vi "json_string_unescape.vi"(11 "escaped string":string) -> (2 "characters unescaped?":bool, 3 "string out":string)   [LabVIEW 2017]
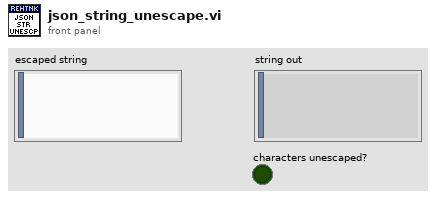
[diagram p1: front panel]
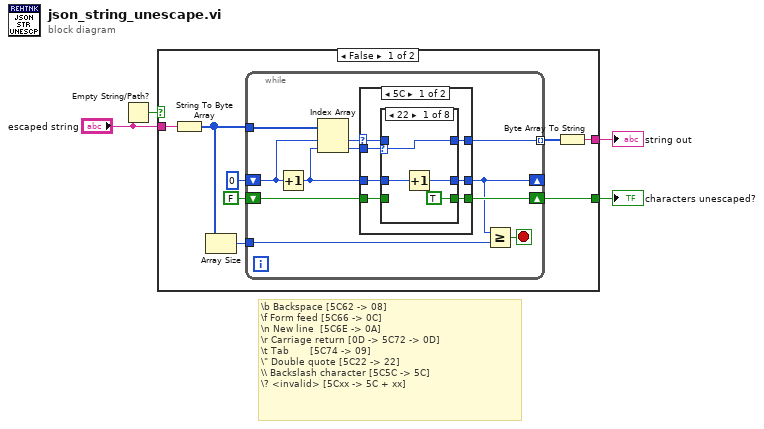
[diagram p0: block diagram]
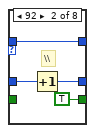
[diagram p2: hidden frame]
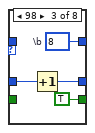
[diagram p3: hidden frame]
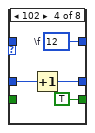
[diagram p4: hidden frame]
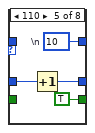
[diagram p5: hidden frame]
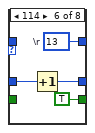
[diagram p6: hidden frame]
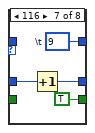
[diagram p7: hidden frame]
diagram:
  # "\\b Backspace [5C62 -> 08]\n\\f Form feed [5C66 -> 0C]\n\\n New line  [5C6E -> 0A]\n\\r Carriage return [0D -> 5C72 -> 0D]\n\\t Tab       [5C74 -> 09]\n\\\" Double quote [5C22 -> 22]\n\\\\ Backslash character [5C5C -> 5C]\n\\? <invalid> [5Cxx -> 5C + xx]"
  n1 = Empty String/Path?(string/path="escaped string") -> (empty?=w1:bool)
  n2 = case shown="False" w1 {
    tunnel: "escaped string" -> [w12 w65]
    tunnel: [w11 _] -> w4
    tunnel: [w8 w65] -> w3
    frame False {
      n3 = String To Byte Array(string=w12) -> (unsigned byte array=w6:u8[])
      n4 = Array Size(array=w6) -> (size(s)=w5:i32)
      n5 = while {
        shift-right: [w20] -> w11
        shift-left: FALSE -> [w19]
        tunnel: [w22] -> w9 mode=indexing
        shift-right: [w16] -> _
        shift-left: 0 -> [w17]
        tunnel: w6 -> [w23]
        tunnel: w5 -> [w15]
        stop <- w14 stop-if-true
        n6 = Increment(x=w17) -> (x+1=w13:i32)
        n7 = Index Array(array=w23, index #1=w17, index #2=w13) -> (element #1=w21:u8, element #2=w18:u8)
        n8 = case shown="5C" w21 {
          selector: w21 -> [w28 w64]
          tunnel: [w29 w64] -> w22
          tunnel: [w25 w63] -> w20
          tunnel: w19 -> [w24 w63]
          tunnel: w18 -> [w30 _]
          tunnel: [w27 w62] -> w16
          tunnel: w13 -> [w26 w62]
          frame 92 {
            n9 = case shown="22" w30 {
              selector: w30 -> [w31 _ _ _ _ _ _ _]
              tunnel: [w31 w38 w40 w44 w48 w52 w56 w61] -> w29
              tunnel: w28 -> [_ w38 _ _ _ _ _ w61]
              tunnel: [w32 w35 w39 w43 w47 w51 w55 w60] -> w27
              tunnel: w26 -> [w34 w37 w42 w46 w50 w54 w58 w60]
              tunnel: [TRUE TRUE TRUE TRUE TRUE TRUE TRUE w59] -> w25
              tunnel: w24 -> [_ _ _ _ _ _ _ w59]
              frame 34 {
                n10 = Increment(x=w34) -> (x+1=w32:i32)
              }
              frame 92 {
                # "\\\\"
                n11 = Increment(x=w37) -> (x+1=w35:i32)
              }
              frame 98 {
                w40 = u8 8  # \b
                n12 = Increment(x=w42) -> (x+1=w39:i32)
              }
              frame 102 {
                w44 = u8 12  # \f
                n13 = Increment(x=w46) -> (x+1=w43:i32)
              }
              frame 110 {
                w48 = u8 10  # \n
                n14 = Increment(x=w50) -> (x+1=w47:i32)
              }
              frame 114 {
                w52 = u8 13  # \r
                n15 = Increment(x=w54) -> (x+1=w51:i32)
              }
              frame 116 {
                w56 = u8 9  # \t
                n16 = Increment(x=w58) -> (x+1=w55:i32)
              }
              frame Default {
              }
            }
          }
          frame Default {
          }
        }
        n17 = Greater Or Equal?(x=w16, y=w15) -> (x >= y?=w14:bool)
      }
      n18 = Byte Array To String(unsigned byte array=w9) -> (string=w8:string)
    }
    frame True {
    }
  }
  "string out" <- w3
  "characters unescaped?" <- w4
